vi "Assemble Module.vi"   [LabVIEW 2021, in "Test VIs.lvclass"]
uses:
  Test VIs/Test VIs.lvclass
  Projects/Sensor Dispense.lvclass
  C:/Users/HEP/Documents/GitHub/Gantry/UCSB-Gantry-HEP-main/Classes/Routine/Dispense/Dispense.lvclass
  Classes/Workspace/Carrier Tray/Assembly Tray.lvclass
  Classes/Controller/Controller.lvclass
  Classes/Controller/Motion/Motion.lvclass
  Classes/Routine/Dispense/Dispense.lvclass
types:
  T1 = typedef "Controller.lvclass/Controllers.ctl" = cluster{"I-O.lvclass":refnum<class "I-O.lvclass">, "Gantry":refnum<k24>, "Dispenser":refnum<visa-resource-name>}
  T2 = typedef "Fixture.lvclass/Workspace.ctl" = cluster{"XYZTheta":dbl[], "Workspace Valve":i32, "Workspace Sensor":i32}
  T3 = cluster{"Motion":dbl[][], "Center":dbl[], "CW/CCW":dbl, "Dispense Type":enum16{"N-gon", "Square", "Arc", "Dot", "Line", "Circle"}}[]
  T4 = enum16{"N-gon", "Square", "Arc", "Dot", "Line", "Circle"}
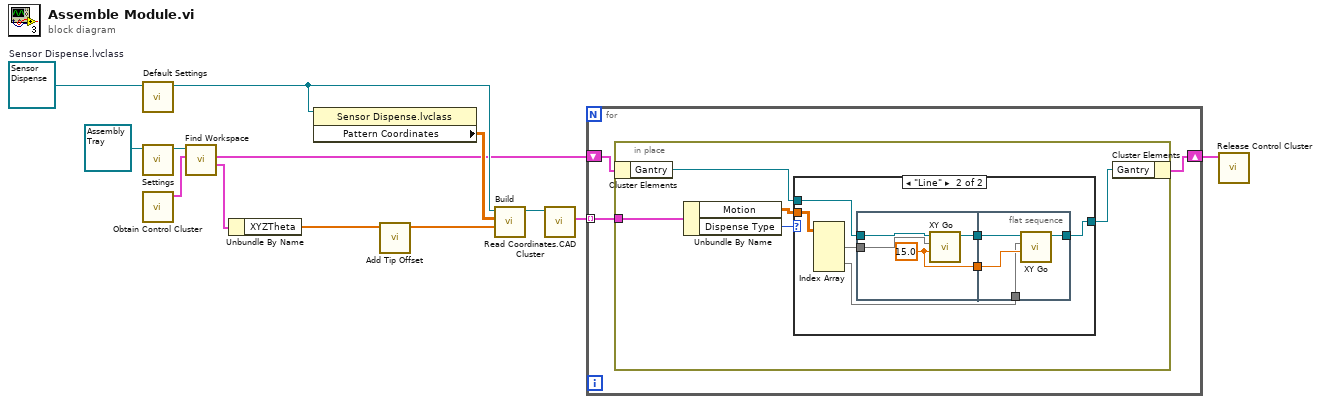
[diagram p0: block diagram]
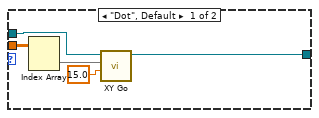
[diagram p2: hidden frame]
diagram:
  w12 = refnum<class "Sensor Dispense.lvclass"> refnum  # Sensor Dispense.lvclass
  n1 = call-dynamic "Default Settings.vi"("Sensor Dispense in"=w12) -> ("Sensor Dispense out"=w11:refnum<class "Sensor Dispense.lvclass">)  [unwired: 9 in, 1 out]
  n2 = call-dynamic "Settings.vi"("Assembly Tray In"=refnum<class "Assembly Tray.lvclass"> refnum ("Assembly Tray.lvclass")) -> ("Assembly Tray Out"=w3:refnum<class "Assembly Tray.lvclass">)  [unwired: 9 in, 1 out]
  n3 = call "Obtain Control Cluster.vi"() -> ("Control Out"=w7:T1)  [unwired: 10 in, 1 out]
  n4 = call-dynamic "Find Workspace.vi"("Control In"=w7, "Carrier Tray in"=w3) -> ("Workspace"=w5:T2, "Control Out"=w6:T1)  [unwired: 6 in, 2 out]
  n5 = Unbundle By Name(w5) -> ("XYZTheta"=w2:dbl[])
  n6 = property class="Sensor Dispense.lvclass"(reference=w11) -> ("Pattern Coordinates"=w10:dbl[][])  [unwired: 1 in, 2 out]
  n7 = call "Add Tip Offset.vi"("XYZTheta"=w2) -> ("XYZTheta"=w1:dbl[])  [unwired: 10 in]
  n8 = call-dynamic "Build.vi"("XYZTheta"=w1, "text file"=w10, "Sensor Dispense in"=w11) -> ("Sensor Dispense out"=w9:refnum<class "Sensor Dispense.lvclass">)  [unwired: 8 in]
  n9 = call-dynamic "Read Coordinates.CAD Cluster.vi"("Sensor Dispense in"=w9) -> ("Coordinates.CAD Cluster"=w8:T3)  [unwired: 8 in, 2 out]
  n10 = for {
    shift-right: [w15] -> w13
    shift-left: w6 -> [w16]
    tunnel: w8 -> [w14] mode=indexing
    n11 = in-place {
      in-place-border: w14 -> [w19]
      n12 = in-place-cluster #1(w16) -> ("Gantry"=w21:refnum<k24>)
      n13 = Unbundle By Name(w19) -> ("Motion"=w17:dbl[][], "Dispense Type"=w18:T4)
      n14 = case shown="\"Line\"" w18 {
        tunnel: w21 -> [w26 w33]
        tunnel: [w25 w32] -> w20
        tunnel: w17 -> [w24 w29]
        frame "Dot", Default {
          n15 = Index Array(array=w24) -> (element=w22:dbl[])  [unwired: 2 in]
          n16 = call "XY Go.vi"("Speed"=15.0, "XY In"=w22, "Gantry In"=w26) -> ("Gantry Out"=w25:refnum<k24>)  [unwired: 6 in, 2 out]
        }
        frame "Line" {
          n17 = Index Array(array=w29) -> (element #1=w28:dbl[], element #2=w27:dbl[])  [unwired: 4 in]
          n18 = flat-sequence {
            tunnel: w33 -> [w37]
            tunnel: [w36] -> w31
            tunnel: [w35] -> w30
            tunnel: w28 -> [w34]
            tunnel: [w40] -> w32
            tunnel: w31 -> [w41]
            tunnel: w30 -> [w39]
            tunnel: w27 -> [w38]
            frame #0 {
              w35 = 15.0 ("Speed")
              n19 = call "XY Go.vi"("Speed"=w35, "XY In"=w34, "Gantry In"=w37) -> ("Gantry Out"=w36:refnum<k24>)  [unwired: 6 in, 2 out]
            }
            frame #1 {
              n20 = call "XY Go.vi"("Speed"=w39, "XY In"=w38, "Gantry In"=w41) -> ("Gantry Out"=w40:refnum<k24>)  [unwired: 6 in, 2 out]
            }
          }
        }
      }
      n21 = in-place-cluster #1("Gantry"=w20) -> (w15:T1)
    }
  }
  n22 = call "Release Control Cluster.vi"("output cluster"=w13) -> ()  [unwired: 11 in]
